vi "Available Images.vi"(8 "error in (no error)":errorcluster, 11 "Refnum in":refnum<k21>) -> (0 "error out":errorcluster, 1 "Images":T1[](array[typedef]) {"component type" items=["standard", "hidden", "system", "unknown", "startup", "image", "essential"]}, 2 "Versions":string[](array[string]), 3 "Refnum out":refnum<k21>)   [LabVIEW 2020]
uses:
  <vilib>/nisyscfg/Software 1.2.ctl
  <vilib>/nisyscfg/Component Type.ctl
  <vilib>/nisyscfg/Get Filtered Base System Images.vi
  <vilib>/nisyscfg/nisyscfg.lvlib
  <resource>/objmgr/nisysapi.rc
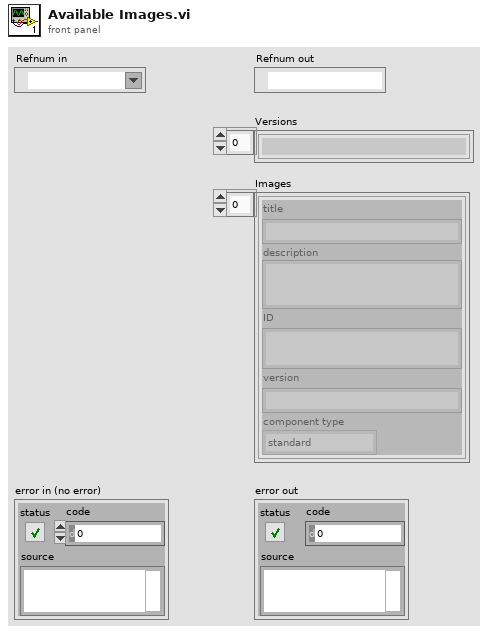
[diagram p1: front panel]
types:
  T1 = typedef "nisyscfg.lvlib/Software 1.2.ctl" = cluster{"title":string, "description":string, "ID":string, "version":string, "component type":T2}
  T2 = typedef "nisyscfg.lvlib/Component Type.ctl" = u32
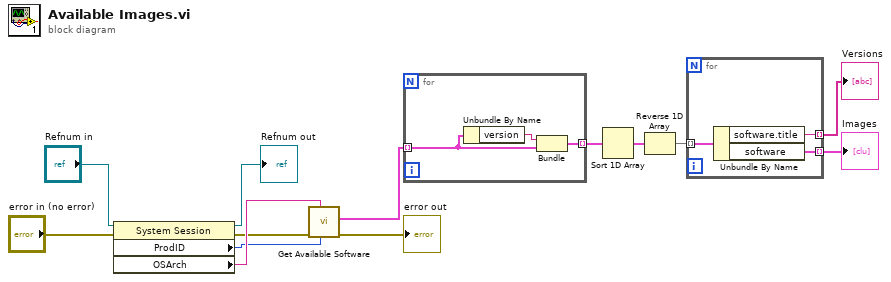
[diagram p0: block diagram]
diagram:
  n1 = property class="System Session"(reference="Refnum in", error in="error in (no error)") -> (reference out=→"Refnum out":refnum<k21>, error out=w8:errorcluster, "ProdID"=w9:i32, "OSArch"=w10:string)
  n2 = call-poly <vilib>:"Get Available Software.vi"("Product ID"=w9, "Operating System"=w10, "error in (no error)"=w8) -> ("error out"=→"error out":errorcluster, "Base System Images"=w3:T1[])  [unwired: 6 in, 1 out]
  n3 = for {
    tunnel: w3 -> [w16] mode=indexing
    tunnel: [w14] -> w4 mode=indexing
    n4 = Unbundle By Name(w16) -> ("version"=w15:string)
    n5 = Bundle("version"=w15, "software"=w16) -> (w14:cluster{"version":string, "software":T1})  [unwired: 1 in]
  }
  n6 = Sort 1D Array(array=w4) -> (sorted array=w5:cluster{"version":string, "software":T1}[])
  n7 = Reverse 1D Array(array=w5) -> (reversed array=w6:cluster{"version":string, "software":T1}[])
  n8 = for {
    tunnel: w6 -> [w19] mode=indexing
    tunnel: [w18] -> w12 mode=indexing
    tunnel: [w17] -> w13 mode=indexing
    n9 = Unbundle By Name(w19) -> ("software.title"=w18:string, "software"=w17:T1)
  }
  "Images" <- w13
  "Versions" <- w12
